vi "send start to orca.vi"(8 "error in (no error)":errorcluster, 11 "Tomo in":refnum<class "Tomo.lvclass">) -> (0 "error out":errorcluster, 3 "Tomo out":refnum<class "Tomo.lvclass">)   [LabVIEW 2012, in "Tomo.lvclass"]
uses:
  Tomo.lvclass
  <vilib>/Distrio/Murmex/StartMessage/StartMessage.lvclass
  <vilib>/Distrio/Murmex/StartMessage/run mode enum.ctl
  Tomo.lvclass/Tomo.ctl
  <vilib>/Distrio/Murmex/Murmex/Murmex.lvclass
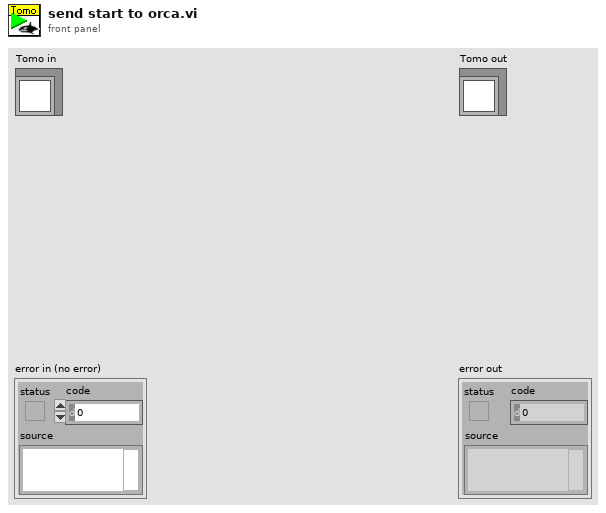
[diagram p1: front panel]
types:
  T1 = typedef "Murmex.lvlib/StartMessage.lvclass/run mode enum.ctl" = enum16{"infinite", "finite"}
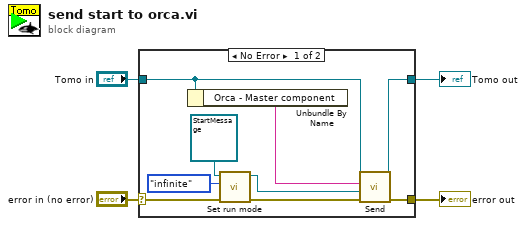
[diagram p0: block diagram]
diagram:
  n1 = case shown="No Error" "error in (no error)" {
    selector: "error in (no error)" -> [w8 w15]
    tunnel: [w13 w15] -> w3
    tunnel: [w10 w14] -> w1
    tunnel: "Tomo in" -> [w11 w14]
    frame No Error {
      n2 = Unbundle By Name(w11) -> ("Orca - Master component"=w12:string)
      n3 = call <vilib>:"Set run mode.vi"("error in (no error)"=w8, "run mode"=run_mode_enum."infinite", "StartMessage in"=refnum<class "StartMessage.lvclass"> refnum ("Message in")) -> ("error out"=w7:errorcluster, "StartMessage out"=w5:refnum<class "StartMessage.lvclass">)  [unwired: 7 in]
      n4 = call <vilib>:"Send.vi"("error in (no error)"=w7, "Message"=w5, "recipient"=w12, "Murmex in"=w11) -> ("error out"=w13:errorcluster, "Murmex out"=w10:refnum<class "Tomo.lvclass">)  [unwired: 6 in]
    }
    frame Error {
    }
  }
  "error out" <- w3
  "Tomo out" <- w1
